vi "1motorVelCtrlTest.vi"() -> ()   [LabVIEW 2020]
uses:
  <vilib>/CISH Robotics/L4VMX TitanQuad/Motor ID.ctl
  <vilib>/Platform/TimedLoop/XDataNode/timing_clust.ctl
  <vilib>/Platform/TimedLoop/XDataNode/nitl_modes.ctl
  <vilib>/Platform/TimedLoop/XDataNode/wakeup.ctl
  <vilib>/CISH Robotics/L4VMX TitanQuad/TitanQuad.lvclass
  <vilib>/platform/TimedLoop/XDataNode/XDataNode.xnode
  <vilib>/Platform/TimedLoop/XDataNode/XDNodeRunTimeDep.lvlib
panel:
  out "error out":errorcluster
  in  "Error In":errorcluster
  out "Finished Late? [i-1]":bool
  out "Waveform Chart":cluster{"Target (deg)":dbl, "Enc (deg)":dbl}(graph)
  in  "reset Encoder":bool
  out "Enc (deg)":dbl
  in  "Motor ID":T1
  in  "Stop Button":bool
  in  "motorSpeed (deg/s)":dbl(slide) scale=-450.0..450.0
  # "M0-M2 「左、右、後輪」 正轉逆時針\nM3 正轉爪向上"
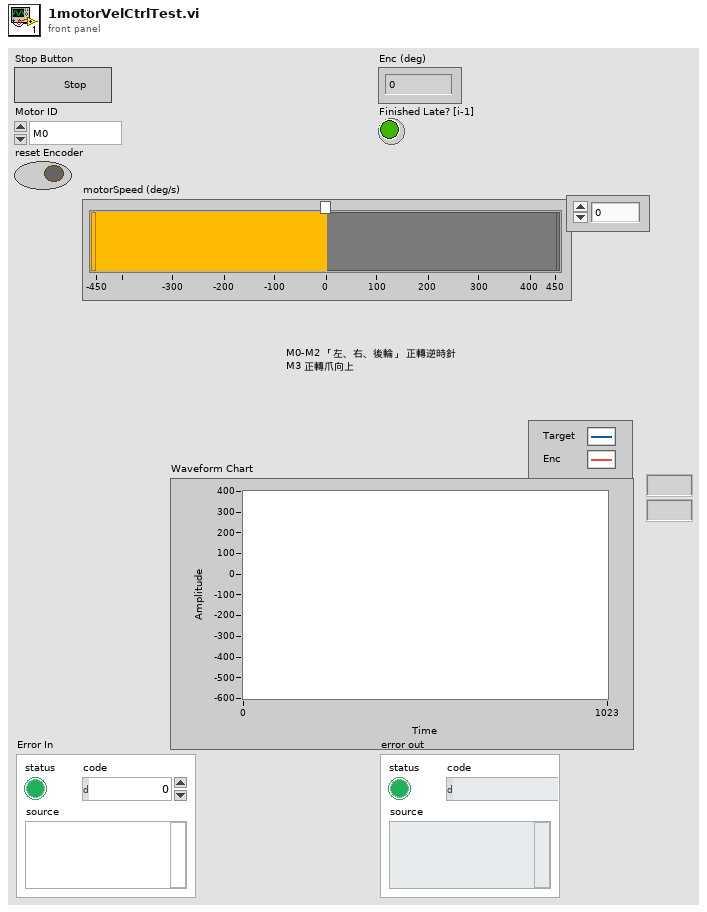
[diagram p1: front panel]
types:
  T1 = typedef "TitanQuad.lvlib/TitanQuad.lvclass/Motor ID.ctl" = enum16{"M0", "M1", "M2", "M3"}
  T2 = typedef "XDNodeRunTimeDep.lvlib/timing_clust.ctl" = cluster{"Expected End [f-1]":u64, "Actual End [f-1]":u64, "Finished Late? [f-1]":bool, "Expected End [i-1]":u64, "Actual End [i-1]":u64, "Finished Late? [i-1]":bool, "Expected Start [i]":u64, "Actual Start [i]":u64, "Expected Start [f]":u64, "Actual Start [f]":u64, "Source Name":string, "Structure Name":string, "Period":i64, "Deadline":i64, "Offset":i64, "Start":i64, "Priority":i32, "Timeout":i32, "Mode":T3, "Wakeup Reason":T4, "Error":errorcluster, "Source Type":string, "Secondary Source Type":string, "Global End Time":u64, "Global Start Time":u64, "Frame Duration":u64, "Iteration Duration":u64, "Assigned CPU":i32, "I/O Scan Engine Mode":u32}
  T3 = typedef "XDNodeRunTimeDep.lvlib/nitl_modes.ctl" = enum32{"No Change", "Process missed periods, maintain original phase", "Discard missed periods, maintain original phase", "Process missed periods, ignore original phase", "Discard missed periods, ignore original phase"}
  T4 = typedef "XDNodeRunTimeDep.lvlib/wakeup.ctl" = enum32{"Normal", "Aborted", "Asynchronous wakeup", "Timing source error", "Timed loop error", "Timeout"}
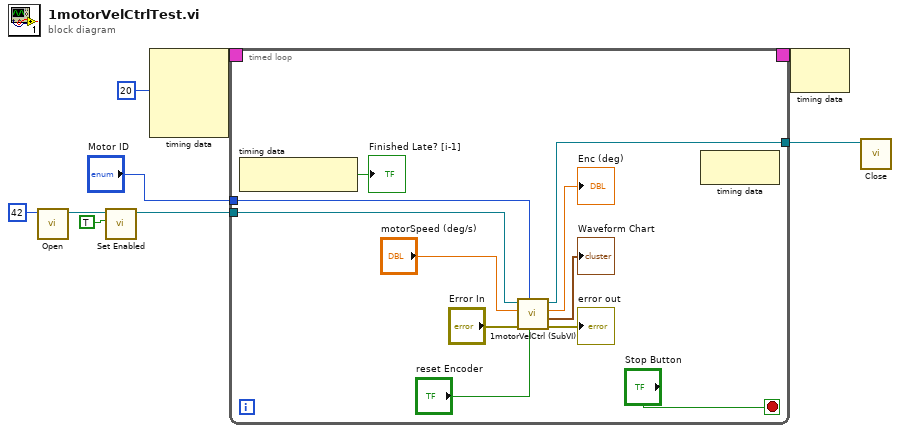
[diagram p0: block diagram]
diagram:
  n1 = call <vilib>:"Open.vi"("Titan ID (42)"=u8 42) -> ("TitanQuad Object"=w9:refnum<class "TitanQuad.lvclass">)  [unwired: 9 in, 1 out]
  n2 = call <vilib>:"Set Enabled.vi"("Enable"=TRUE, "TitanQuad Object"=w9) -> ("TitanQuad Object"=w8:refnum<class "TitanQuad.lvclass">)  [unwired: 8 in, 1 out]
  n3 = node-c288(i64 20 ("Period")) -> (w3:T2)  [unwired: 3 in]
  n4 = timed-loop {
    tunnel: w8 -> [w18]
    tunnel: [w20] -> w7
    tunnel: "Motor ID" -> [w12]
    timing: w3 -> [_]
    timing-out: [_] -> w2
    stop <- "Stop Button" stop-if-true
    n5 = node-c288() -> (→"Finished Late? [i-1]":bool)  [unwired: 1 in]
    n6 = call "1motorVelCtrl (SubVI).vi"("reset Encoder"="reset Encoder", "Motor ID"=w12, "error in (no error)"="Error In", "motorSpeed (deg/s)"="motorSpeed (deg/s)", "TitanQuad in"=w18) -> ("error out"=→"error out":errorcluster, "Cluster"=→"Waveform Chart":cluster{"Target (deg)":dbl, "Enc (deg)":dbl}, "Enc (deg)"=→"Enc (deg)":dbl, "TitanQuad out"=w20:refnum<class "TitanQuad.lvclass">)  [unwired: 3 in]
    n7 = node-c288() -> ()  [unwired: 1 in, 1 out]
  }
  n8 = node-c288(w2) -> ()  [unwired: 1 out]
  n9 = call <vilib>:"Close.vi"("TitanQuad Object"=w7) -> ()  [unwired: 10 in, 1 out]
